vi "Read Dashboard Variables.vi"() -> ()   [LabVIEW 2018]
uses:
  <vilib>/Rock Robotics/Network Tables/NT Read Number.vi
  Framework/Robot Global Data.vi
panel:
  out "Cargo Stop Current":dbl
  out "Cargo Hold Duration":dbl
  out "Cheezy Drive Mode":u32=2
  out "Cargo Setpoint":dbl
  out "Elevator Duration":dbl
  out "Elevator Setpoint":dbl
  out "Pivot Right Setpoint":dbl
  out "Pivot Left Setpoint":dbl
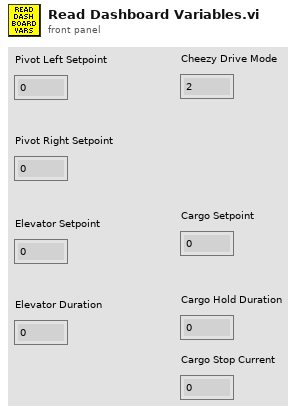
[diagram p1: front panel]
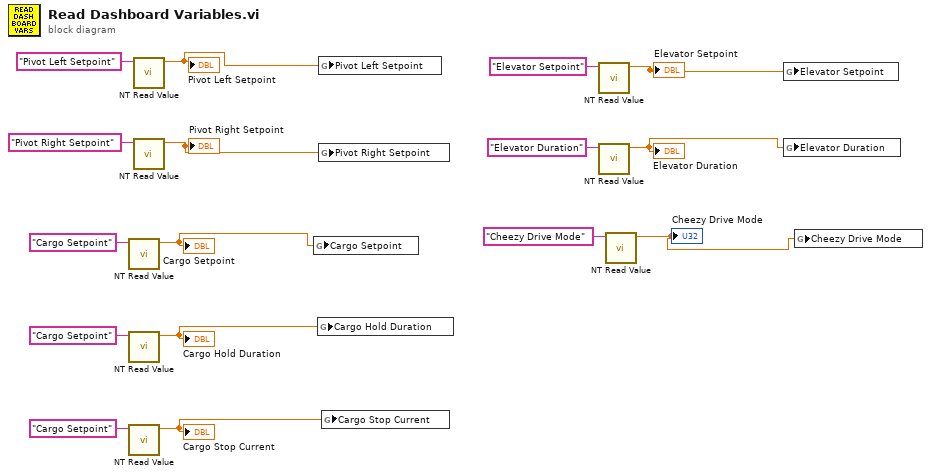
[diagram p0: block diagram]
diagram:
  n1 = call-poly <vilib>:"NT Read Value.vi"("Name"="Cargo Setpoint") -> ("Numeric"=w6:dbl)  [unwired: 9 in, 1 out]
  "Cargo Setpoint" <- w6
  n2 = call-poly <vilib>:"NT Read Value.vi"("Name"="Cargo Setpoint") -> ("Numeric"=w4:dbl)  [unwired: 9 in, 1 out]
  "Cargo Hold Duration" <- w4
  n3 = call-poly <vilib>:"NT Read Value.vi"("Name"="Cargo Setpoint") -> ("Numeric"=w1:dbl)  [unwired: 9 in, 1 out]
  "Cargo Stop Current" <- w1
  n4 = call-poly <vilib>:"NT Read Value.vi"("Name"="Pivot Left Setpoint") -> ("Numeric"=w10:dbl)  [unwired: 9 in, 1 out]
  "Pivot Left Setpoint" <- w10
  n5 = call-poly <vilib>:"NT Read Value.vi"("Name"="Pivot Right Setpoint") -> ("Numeric"=w9:dbl)  [unwired: 9 in, 1 out]
  "Pivot Right Setpoint" <- w9
  n6 = global write "Robot Global Data.vi" "Cargo Setpoint"(w6) -> ()
  n7 = global write "Robot Global Data.vi" "Cargo Hold Duration"(w4) -> ()
  n8 = global write "Robot Global Data.vi" "Pivot Left Setpoint"(w10) -> ()
  n9 = global write "Robot Global Data.vi" "Pivot Right Setpoint"(w9) -> ()
  n10 = global write "Robot Global Data.vi" "Cargo Stop Current"(w1) -> ()
  n11 = call-poly <vilib>:"NT Read Value.vi"("Name"="Elevator Setpoint") -> ("Numeric"=w8:dbl)  [unwired: 9 in, 1 out]
  "Elevator Setpoint" <- w8
  n12 = call-poly <vilib>:"NT Read Value.vi"("Name"="Elevator Duration") -> ("Numeric"=w7:dbl)  [unwired: 9 in, 1 out]
  "Elevator Duration" <- w7
  n13 = call-poly <vilib>:"NT Read Value.vi"("Name"="Cheezy Drive Mode") -> ("Numeric"=w5:dbl)  [unwired: 9 in, 1 out]
  "Cheezy Drive Mode" <- w5
  n14 = global write "Robot Global Data.vi" "Elevator Setpoint"(w8) -> ()
  n15 = global write "Robot Global Data.vi" "Elevator Duration"(w7) -> ()
  n16 = global write "Robot Global Data.vi" "Cheezy Drive Mode"(w5) -> ()
